vi "Lognormal Inverse CDF.vi"(9 "c":dbl=3.0, 10 "b":dbl=2.0, 11 "cdf(x)":dbl=0.40863834423098205) -> (0 "error":i32, 3 "x":dbl=1.000000005)   [LabVIEW 2010, in "NI_Gmath.lvlib"]
doc: "Computes the continuous inverse cumulative distribution function (CDF) of the various distributions. You must manually select the polymorphic instance to use."
uses:
  NI_Gmath.lvlib
  st_error_code.ctl
panel:
  # "Lognormal Inverse CDF"
  # "median (scale)"
  # "standard dev (shape)"
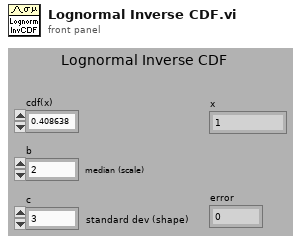
[diagram p1: front panel]
types:
  T1 = typedef "NI_Gmath.lvlib/st_error_code.ctl" = i32
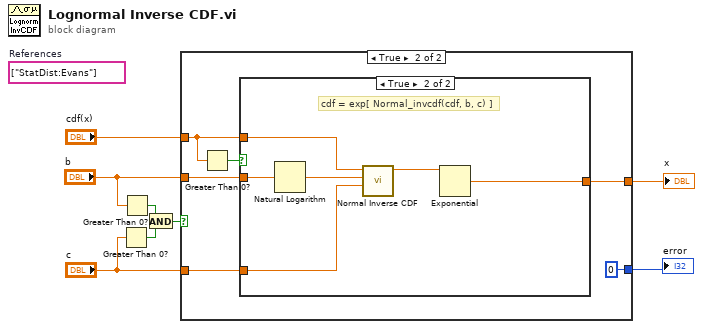
[diagram p0: block diagram]
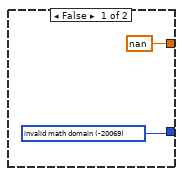
[diagram p2: hidden frame]
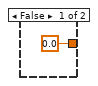
[diagram p3: hidden frame]
diagram:
  (unwired) string[] ["StatDist:Evans"]  # References
  n1 = Greater Than 0?(x="c") -> (x > 0?=w6:bool)
  n2 = Greater Than 0?(x="b") -> (x > 0?=w7:bool)
  n3 = And(x=w7, y=w6) -> (x .and. y?=w8:bool)
  n4 = case shown="True" w8 {
    tunnel: "c" -> [_ w13]
    tunnel: [w9 0 ("invalid math domain")] -> w1
    tunnel: [nan w14] -> w2
    tunnel: "cdf(x)" -> [_ w11]
    tunnel: "b" -> [_ w15]
    frame False {
      w9 = T1 -20069 items=["invalid math domain"=-20069, "Fourier interpolation size m >= n"=-20070, "empty array"=-20003] ("stat interp error code")
    }
    frame True {
      n5 = Greater Than 0?(x=w11) -> (x > 0?=w12:bool)
      n6 = case shown="True" w12 {
        tunnel: w15 -> [_ w19]
        tunnel: [0.0 w20] -> w14
        tunnel: w11 -> [_ w23]
        tunnel: w13 -> [_ w22]
        frame False {
        }
        frame True {
          # "cdf = exp[ Normal_invcdf(cdf, b, c) ]"
          n7 = Natural Logarithm(1:w19) -> (0:w18:dbl)
          n8 = call "Normal Inverse CDF.vi"("std"=w22, "mean"=w18, "cdf(x)"=w23) -> ("x"=w21:dbl)  [unwired: 7 in, 1 out]
          n9 = Exponential(1:w21) -> (0:w20:dbl)
        }
      }
    }
  }
  "x" <- w2
  "error" <- w1
